vi "Playback Frame Cropping.vi"(8 "error in (no error)":errorcluster, 11 "Frame Grabber Data in":T2={"Camera Session"="", "Frame"=refnum, "AVI Refnum"=refnum, "Codecs"=[], "Frame number"=0, "Tracking File Refnum"=refnum, "Tick Count"=0, "Probe Object"=refnum, "Playback Probe Data"=[], "Rigid Body"={"Position"={"x (mm)"=0.0, "y (mm)"=0.0, "z (mm)"=0.0}, "Orientation"={"Pitch (rad)"=0.0, "Yaw (rad)"=0.0, "Roll (rad)"=0.0}, "Quaternion"={"qx"=0.0, "qy"=0.0, "qz"=0.0, "qw"=0.0}, "Tracked?"=FALSE}, "Total no frames playback"=0, "Video FPS"=0.0, "Camera connected?"=FALSE, "Scene"=refnum, "Cropped Frame"=refnum, "Tracker FPS"=0.0, "Crop ROI"=[], "Presentation Values"=[], "Elapsed time (ms)"=0, "Camera frames playback"=0, "Refnums"={"Live Refnum"=refnum, "Record Refnum"=refnum, "Recording Settings Refnum"=refnum, "Playback Refnum"=refnum, "Frame Slider Refnum"=refnum, "Pause Refnum"=refnum, "Home Refnum"=refnum, "Crop Refnum"=refnum, "Clear Crop Refnum"=refnum, "stop refnum"=refnum, "Playback Rate Refnum"=refnum, "Operator Settings Refnums"=refnum, "Presentation Refnum"=refnum, "Gestation Refnum"=refnum, "Connection Settings Refnum"=refnum, "Crop Time Frame Slider Refnum"=refnum}, "Dimensions"={"Probe Dimensions"={"Probe Width"=0.0, "Probe Depth"=1.0, "Probe Height"=0.0}, "Room Dimensions"={"Room Width"=0.0, "Room Depth"=0.0, "Room Height"=0.0}}, "Playback Data As Strings"=[], "Cropped Tracking File Refnum"=refnum, "Cropped AVI Refnum"=refnum, "Header"=[]}) -> (0 "error out":errorcluster, 1 "Continue playback?":bool, 2 "Image":T1, 3 "Frame Grabber Data out":T2={"Camera Session"="", "Frame"=refnum, "AVI Refnum"=refnum, "Codecs"=[], "Frame number"=0, "Tracking File Refnum"=refnum, "Tick Count"=0, "Probe Object"=refnum, "Playback Probe Data"=[], "Rigid Body"={"Position"={"x (mm)"=0.0, "y (mm)"=0.0, "z (mm)"=0.0}, "Orientation"={"Pitch (rad)"=0.0, "Yaw (rad)"=0.0, "Roll (rad)"=0.0}, "Quaternion"={"qx"=0.0, "qy"=0.0, "qz"=0.0, "qw"=0.0}, "Tracked?"=FALSE}, "Total no frames playback"=0, "Video FPS"=0.0, "Camera connected?"=FALSE, "Scene"=refnum, "Cropped Frame"=refnum, "Tracker FPS"=0.0, "Crop ROI"=[], "Presentation Values"=[], "Elapsed time (ms)"=0, "Camera frames playback"=0, "Refnums"={"Live Refnum"=refnum, "Record Refnum"=refnum, "Recording Settings Refnum"=refnum, "Playback Refnum"=refnum, "Frame Slider Refnum"=refnum, "Pause Refnum"=refnum, "Home Refnum"=refnum, "Crop Refnum"=refnum, "Clear Crop Refnum"=refnum, "stop refnum"=refnum, "Playback Rate Refnum"=refnum, "Operator Settings Refnums"=refnum, "Presentation Refnum"=refnum, "Gestation Refnum"=refnum, "Connection Settings Refnum"=refnum, "Crop Time Frame Slider Refnum"=refnum}, "Dimensions"={"Probe Dimensions"={"Probe Width"=0.0, "Probe Depth"=1.0, "Probe Height"=0.0}, "Room Dimensions"={"Room Width"=0.0, "Room Depth"=0.0, "Room Height"=0.0}}, "Playback Data As Strings"=[], "Cropped Tracking File Refnum"=refnum, "Cropped AVI Refnum"=refnum, "Header"=[]}, 5 "Camera frame number":u32)   [LabVIEW 2017]
uses:
  Controls/Frame Grabber Data.ctl
  <vilib>/userdefined/High Color/IMAQdx.ctl
  <vilib>/vision/Image Controls.llb/IMAQ Image.ctl
  <vilib>/vision/Avi.llb/IMAQ AVI2 Refnum.ctl
  Controls/Rigid Body Info.ctl
  Controls/Position.ctl
  Controls/Orientation.ctl
  Controls/Refnums.ctl
  Controls/Recording Settings.ctl
  Controls/Operator Settings.ctl
  Controls/Operator.ctl
  Controls/Dimensions.ctl
  Controls/Room Dimensions.ctl
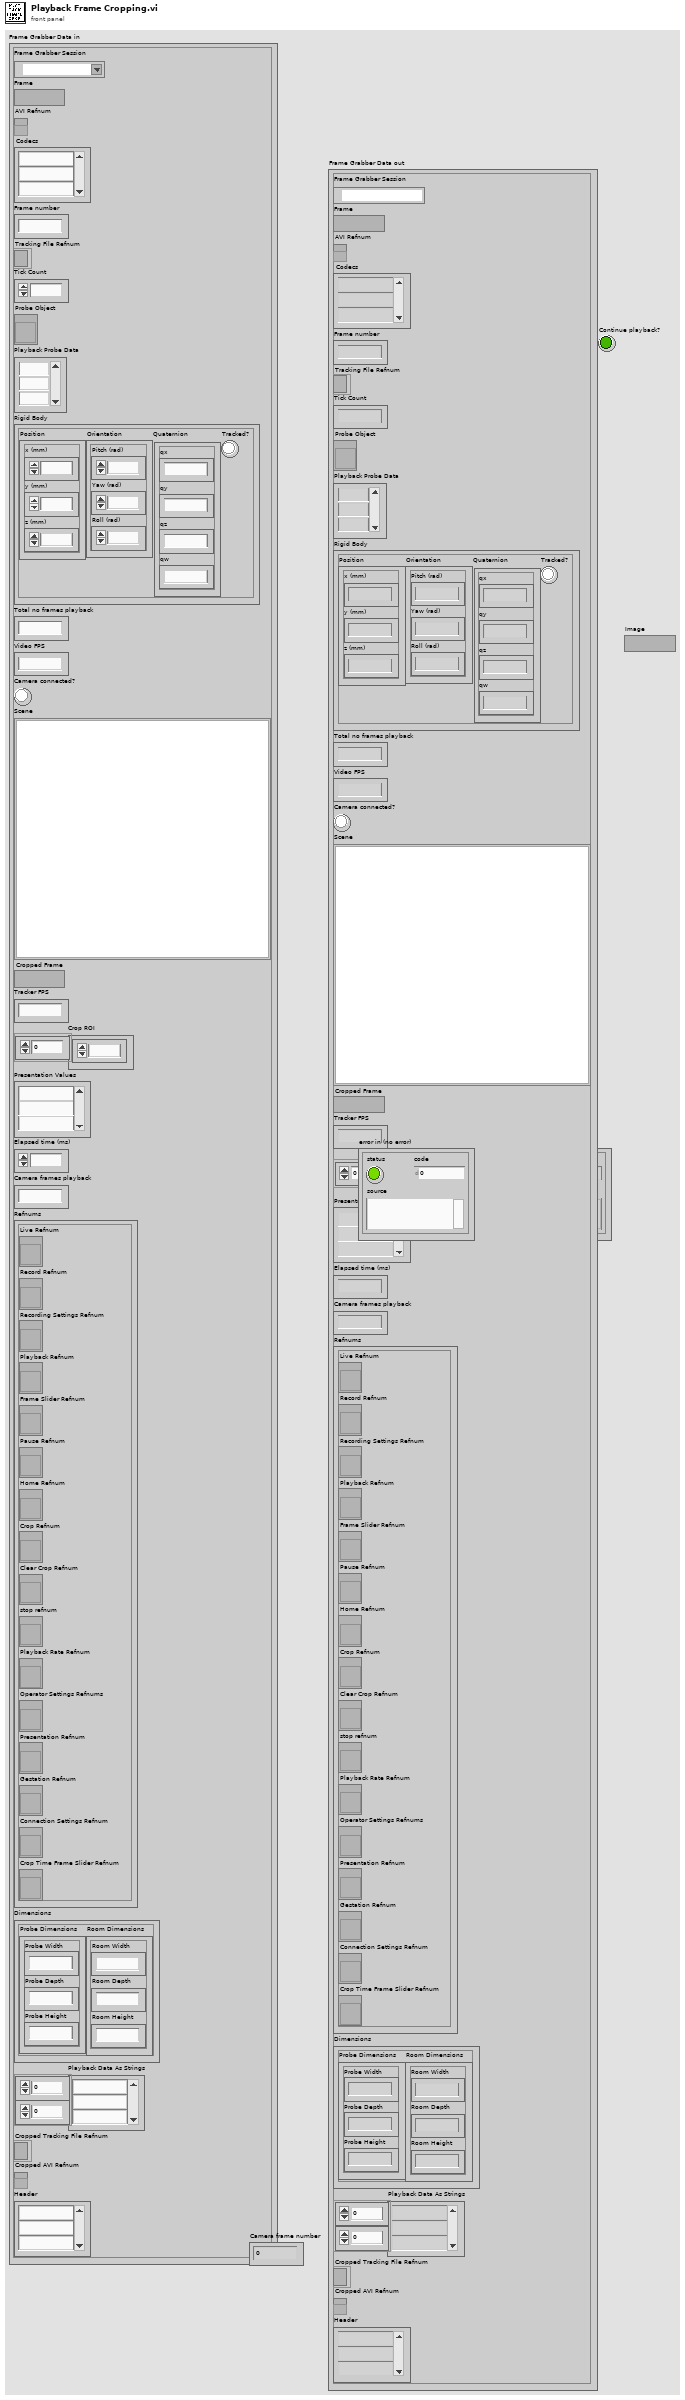
[diagram p1: front panel]
types:
  T1 = typedef "IMAQ Image.ctl" = refnum<image>
  T2 = typedef "Frame Grabber Data.ctl" = cluster{"Camera Session":T3, "Frame":T1, "AVI Refnum":T4, "Codecs":string[], "Frame number":u32, "Tracking File Refnum":refnum<file>, "Tick Count":u32, "Probe Object":refnum<vi>, "Playback Probe Data":dbl[][], "Rigid Body":T5, "Total no frames playback":i32, "Video FPS":dbl, "Camera connected?":bool, "Scene":refnum<vi>, "Cropped Frame":T1, "Tracker FPS":dbl, "Crop ROI":i32[], "Presentation Values":string[], "Elapsed time (ms)":u32, "Camera frames playback":u32, "Refnums":T8, "Dimensions":T9, "Playback Data As Strings":string[][], "Cropped Tracking File Refnum":refnum<file>, "Cropped AVI Refnum":T4, "Header":string[]}
  T3 = typedef "IMAQdx.ctl" = refnum<k21>
  T4 = typedef "IMAQ AVI2 Refnum.ctl" = refnum<k20>
  T5 = typedef "Rigid Body Info.ctl" = cluster{"Position":T6, "Orientation":T7, "Quaternion":cluster{"qx":sgl, "qy":sgl, "qz":sgl, "qw":sgl}, "Tracked?":bool}
  T6 = typedef "Position.ctl" = cluster{"x (mm)":sgl, "y (mm)":sgl, "z (mm)":sgl}
  T7 = typedef "Orientation.ctl" = cluster{"Pitch (rad)":sgl, "Yaw (rad)":sgl, "Roll (rad)":sgl}
  T8 = typedef "Refnums.ctl" = cluster{"Live Refnum":refnum<vi>, "Record Refnum":refnum<vi>, "Recording Settings Refnum":refnum<vi>, "Playback Refnum":refnum<vi>, "Frame Slider Refnum":refnum<vi>, "Pause Refnum":refnum<vi>, "Home Refnum":refnum<vi>, "Crop Refnum":refnum<vi>, "Clear Crop Refnum":refnum<vi>, "stop refnum":refnum<vi>, "Playback Rate Refnum":refnum<vi>, "Operator Settings Refnums":refnum<vi>, "Presentation Refnum":refnum<vi>, "Gestation Refnum":refnum<vi>, "Connection Settings Refnum":refnum<vi>, "Crop Time Frame Slider Refnum":refnum<vi>}
  T9 = typedef "Dimensions.ctl" = cluster{"Probe Dimensions":cluster{"Probe Width":sgl, "Probe Depth":sgl, "Probe Height":sgl}, "Room Dimensions":T10}
  T10 = typedef "Room Dimensions.ctl" = cluster{"Room Width":dbl, "Room Depth":dbl, "Room Height":dbl}
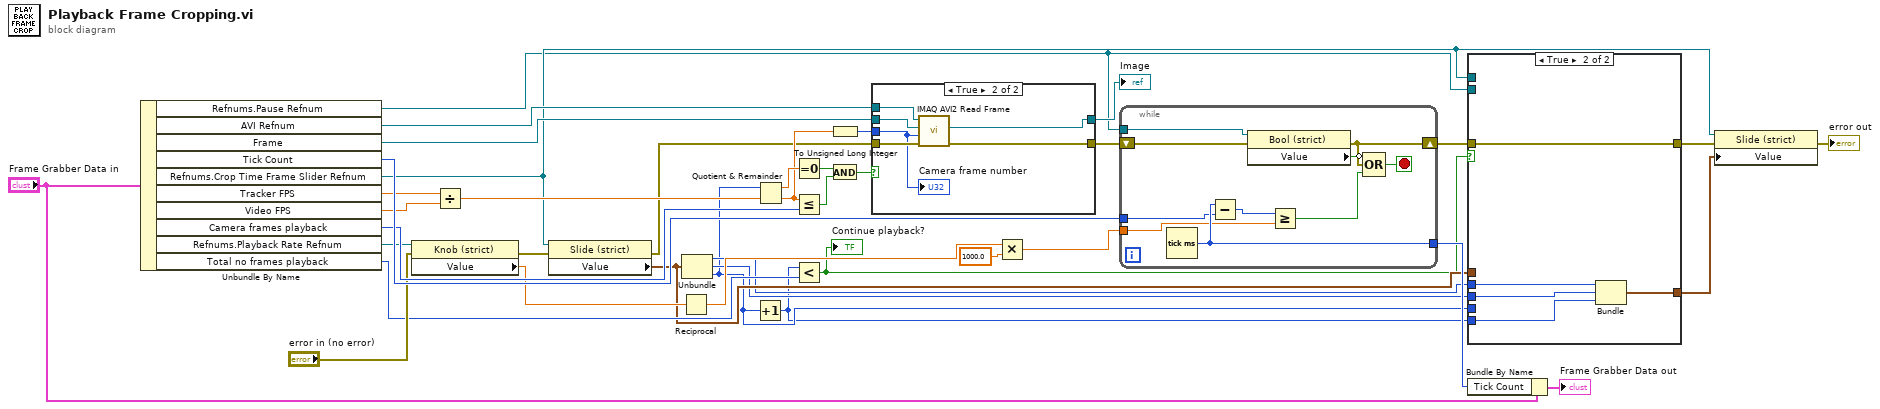
[diagram p0: block diagram]
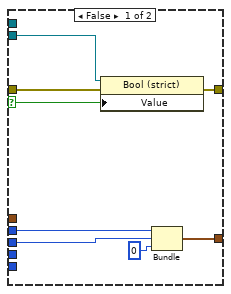
[diagram p2: hidden frame]
diagram:
  n1 = Unbundle By Name("Frame Grabber Data in") -> ("Refnums.Pause Refnum"=w8:refnum<vi>, "AVI Refnum"=w37:T4, "Frame"=w38:T1, "Tick Count"=w31:u32, "Refnums.Crop Time Frame Slider Refnum"=w12:refnum<vi>, "Tracker FPS"=w28:dbl, "Video FPS"=w27:dbl, "Camera frames playback"=w24:u32, "Refnums.Playback Rate Refnum"=w16:refnum<vi>, "Total no frames playback"=w15:i32)
  n2 = property class="Knob (strict)"(reference=w16, error in="error in (no error)") -> (error out=w17:errorcluster, "Value"=w19:dbl)  [unwired: 1 out]
  n3 = Divide(x=w28, y=w27) -> (x/y=w26:dbl)
  n4 = property class="Slide (strict)"(reference=w12, error in=w17) -> (error out=w21:errorcluster, "Value"=w11:cluster{i32, i32, i32})  [unwired: 1 out]
  n5 = Reciprocal(x=w19) -> (1/x=w34:dbl)
  n6 = Unbundle(w11) -> (w5:i32, w4:i32, w3:i32)
  n7 = Increment(x=w3) -> (x+1=w2:i32)
  n8 = Quotient & Remainder(x=w3, y=w26) -> (x-y*floor(x/y)=w30:dbl, floor(x/y)=w25:dbl)
  n9 = Equal To 0?(x=w30) -> (x = 0?=w29:bool)
  n10 = Less Or Equal?(x=w25, y=w24) -> (x <= y?=w22:bool)
  n11 = Less?(x=w2, y=w15) -> (x < y?=w9:bool)
  "Continue playback?" <- w9
  n12 = To Unsigned Long Integer(number=w25) -> (unsigned 32bit integer=w14:u32)
  n13 = And(x=w29, y=w22) -> (x .and. y?=w23:bool)
  n14 = case shown="True" w23 {
    tunnel: [w40 w47] -> w39
    tunnel: w38 -> [w40 w46]
    tunnel: w37 -> [_ w45]
    tunnel: [w41 w44] -> w20
    tunnel: w21 -> [w41 w43]
    tunnel: w14 -> [_ w42]
    frame False {
    }
    frame True {
      n15 = call "IMAQ AVI2 Read Frame"("error in (no error)"=w43, "Frame Number"=w42, "Image"=w46, "AVI Refnum"=w45) -> ("error out"=w44:errorcluster, "Image Out"=w47:T1)  [unwired: 5 in, 1 out]
      "Camera frame number" <- w42
    }
  }
  "Image" <- w39
  n16 = Multiply(x=w34, y=1000.0) -> (x*y=w32:dbl)
  n17 = while {
    tunnel: [w57] -> w35
    tunnel: w32 -> [w55]
    tunnel: w31 -> [w54]
    shift-right: [w50] -> w13
    shift-left: w20 -> [w51]
    tunnel: w8 -> [w49]
    stop <- w53 stop-if-true
    n18 = Tick Count (ms)() -> (millisecond timer value=w57:u32)
    n19 = Subtract(x=w57, y=w54) -> (x-y=w56:u32)
    n20 = property class="Bool (strict)"(reference=w49, error in=w51) -> (error out=w50:errorcluster, "Value"=w48:bool)  [unwired: 1 out]
    n21 = Greater Or Equal?(x=w56, y=w55) -> (x >= y?=w52:bool)
    n22 = Compound Arithmetic op=OR(invert w48, w50, w52) -> (w53:bool)
  }
  n23 = case shown="True" w9 {
    selector: w9 -> [w63 _]
    tunnel: w13 -> [w59 w66]
    tunnel: w12 -> [_ _]
    tunnel: w11 -> [_ _]
    tunnel: w8 -> [w64 _]
    tunnel: [w62 w70] -> w7
    tunnel: w5 -> [w61 w69]
    tunnel: w4 -> [w60 w68]
    tunnel: w3 -> [_ _]
    tunnel: w2 -> [_ w67]
    tunnel: [w58 w66] -> w1
    frame False {
      n24 = property class="Bool (strict)"(reference=w64, error in=w59, "Value"=w63) -> (error out=w58:errorcluster)  [unwired: 1 out]
      n25 = Bundle(w61, w60, u32 0) -> (w62:cluster{i32, i32, u32})  [unwired: 1 in]
    }
    frame True {
      n26 = Bundle(w69, w68, w67) -> (w70:cluster{i32, i32, i32})  [unwired: 1 in]
    }
  }
  n27 = Bundle By Name(cluster="Frame Grabber Data in", "Tick Count"=w35) -> (→"Frame Grabber Data out":T2)
  n28 = property class="Slide (strict)"(reference=w12, error in=w1, "Value"=w7) -> (error out=→"error out":errorcluster)  [unwired: 1 out]
